vi "MonoList.vi"(8 "error in (no error)":errorcluster, 10 "Delay between send and receive [ms]":i32=5000, 11 "Communicator in":refnum<class "Communicator.lvclass">) -> (0 "error out":errorcluster, 1 "ID":i32, 2 "results-JSON":string, 3 "Communicator out":refnum<class "Communicator.lvclass">)   [LabVIEW 2023, in "DeviceManager.lvlib"]
uses:
  Libraries/DeviceManager/DeviceManager.lvlib
  Communicator/Communicator.lvclass
panel:
  # "Connector Pane"
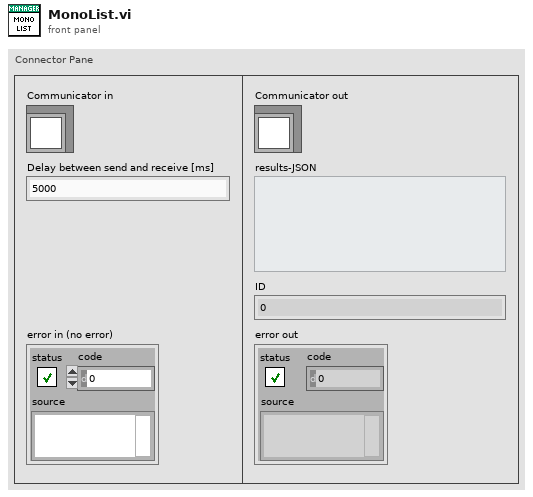
[diagram p1: front panel]
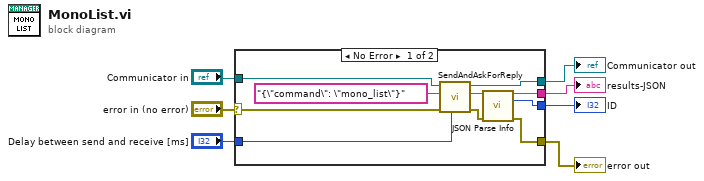
[diagram p0: block diagram]
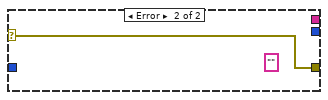
[diagram p2: hidden frame]
diagram:
  n1 = case shown="No Error" "error in (no error)" {
    selector: "error in (no error)" -> [w16 w18]
    tunnel: [w11 w18] -> w6
    tunnel: "Delay between send and receive [ms]" -> [w17 _]
    tunnel: [w12 _] -> w4
    tunnel: [w10 _] -> w3
    tunnel: "Communicator in" -> [w9 _]
    tunnel: [w8 _] -> w1
    frame No Error {
      n2 = call-dynamic "SendAndAskForReply.vi"("Delay between send and receive [ms]"=w17, "error in (no error)"=w16, "String to be sent"="{\"command\": \"mono_list\"}", "Communicator in"=w9) -> ("error out"=w13:errorcluster, "Data"=w14:string, "Communicator out"=w8:refnum<class "Communicator.lvclass">)  [unwired: 5 in]
      n3 = call "JSON Parse Info.vi"("JSON"=w14, "error in (no error)"=w13) -> ("results-JSON"=w10:string, "ID"=w12:i32, "error out"=w11:errorcluster)  [unwired: 11 in]
    }
    frame Error {
      (unwired) "" ("<JSON>")
    }
  }
  "error out" <- w6
  "ID" <- w4
  "results-JSON" <- w3
  "Communicator out" <- w1
